vi "WriteNodeIDtoSettings.vi"(0 "File Path In":path, 5 "OPCUA Setting In":T1, 7 "NodeID In":string, 11 "error in (no error)":errorcluster) -> (4 "OK":bool, 15 "error out":errorcluster)   [LabVIEW 2024, in "OPCUA.lvlib"]
uses:
  OPCUA.lvlib
  OPCUA Setting.ctl
  <vilib>/Utility/xml.llb/Write to XML File(string).vi
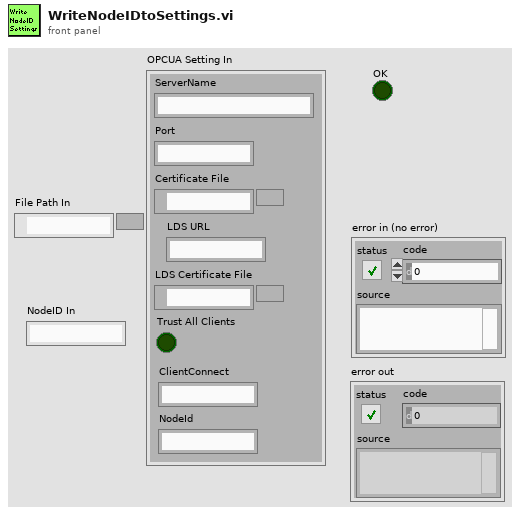
[diagram p1: front panel]
types:
  T1 = typedef "OPCUA.lvlib/OPCUA Setting.ctl" = cluster{"ServerName":string, "Port":string, "Certificate File":path, "LDS URL":string, "LDS Certificate File":path, "Trust All Clients":bool, "ClientConnect":string, "NodeId":string}
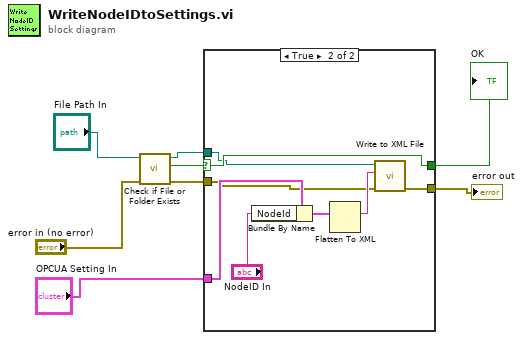
[diagram p0: block diagram]
diagram:
  n1 = call <vilib>:"Check if File or Folder Exists.vi"("error in (no error)"="error in (no error)", "path"="File Path In") -> ("error out"=w3:errorcluster, "file or folder exists?"=w5:bool, "dup path"=w4:path)  [unwired: 7 in]
  n2 = case shown="True" w5 {
    selector: w5 -> [w10 w14]
    tunnel: [w9 w15] -> w7
    tunnel: [w10 w14] -> w6
    tunnel: w4 -> [_ w12]
    tunnel: w3 -> [w9 w11]
    tunnel: "OPCUA Setting In" -> [_ w13]
    frame False {
    }
    frame True {
      n3 = Bundle By Name(cluster=w13, "NodeId"="NodeID In") -> (w17:T1)
      n4 = Flatten To XML(6:w17) -> (2:w16:string)
      n5 = call-poly <vilib>:"Write to XML File.vi"("error in (no error)"=w11, "XML Input"=w16, "XML File Path"=w12) -> ("error out"=w15:errorcluster)  [unwired: 6 in, 2 out]
    }
  }
  "error out" <- w7
  "OK" <- w6
